vi "Error Checking.vi"(8 "error in (no error)":errorcluster, 11 "VISA resource name":refnum<visa-resource-name>) -> (0 "error out":errorcluster, 2 "Connection Error":bool, 3 "VISA resource name":refnum<visa-resource-name>)   [LabVIEW 2018]
uses:
  <vilib>/Utility/error.llb/DialogType.ctl
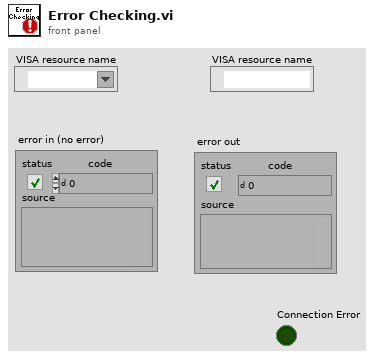
[diagram p1: front panel]
types:
  T1 = typedef "DialogType.ctl" = u16
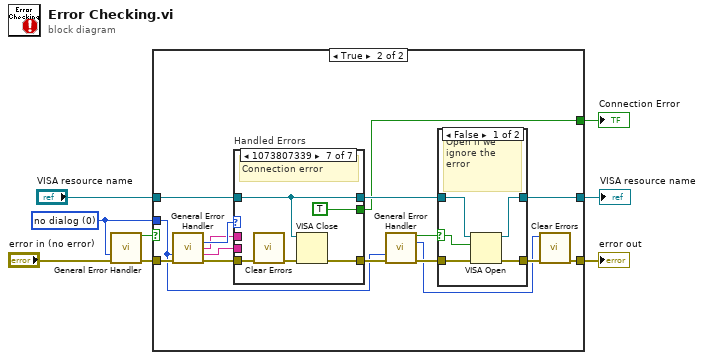
[diagram p0: block diagram]
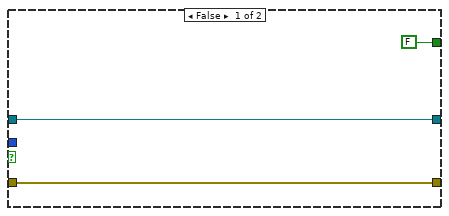
[diagram p2: hidden frame]
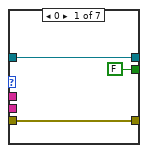
[diagram p4: hidden frame]
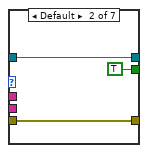
[diagram p5: hidden frame]
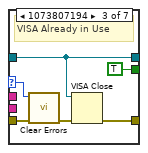
[diagram p6: hidden frame]
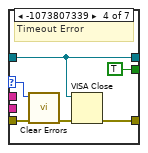
[diagram p7: hidden frame]
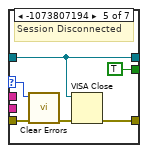
[diagram p8: hidden frame]
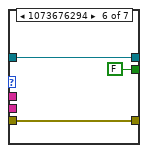
[diagram p9: hidden frame]
diagram:
  w2 = T1 0 items=["no dialog", "OK message", "continue or stop message", "OK message + warnings", "continue/stop + warnings"] ("type of dialog (OK msg:1)")
  n1 = call <vilib>:"General Error Handler.vi"("type of dialog (OK msg:1)"=w2, "error in (no error)"="error in (no error)") -> ("error?"=w8:bool, "error out"=w7:errorcluster)  [unwired: 9 in, 3 out]
  n2 = case shown="True" w8 {
    tunnel: [w11 w26] -> w6
    tunnel: w7 -> [w11 w27]
    tunnel: "VISA resource name" -> [w10 w25]
    tunnel: [w10 w19] -> w3
    tunnel: w2 -> [_ w17]
    tunnel: [FALSE w12] -> w1
    frame False {
    }
    frame True {
      n3 = call <vilib>:"General Error Handler.vi"("type of dialog (OK msg:1)"=w17, "error in (no error)"=w27) -> ("code out"=w15:i32, "source out"=w14:string, "message"=w13:string, "error out"=w24:errorcluster)  [unwired: 9 in, 1 out]
      n4 = case "Handled Errors" shown="1073807339" w15 {
        selector: w15 -> [_ _ w42 w48 w54 _ _]
        tunnel: w24 -> [w37 w40 w44 w50 w56 w61 w65]
        tunnel: [w37 w40 w46 w52 w58 w61 w63] -> w23
        tunnel: w14 -> [_ _ _ _ _ _ _]
        tunnel: w13 -> [_ _ _ _ _ _ _]
        tunnel: w25 -> [w36 w39 w45 w51 w57 w60 w64]
        tunnel: [w36 w39 w45 w51 w57 w60 w64] -> w18
        tunnel: [FALSE TRUE TRUE TRUE TRUE FALSE TRUE] -> w12
        frame 0 {
        }
        frame Default {
        }
        frame 1073807194 {
          # "VISA Already in Use"
          n5 = call <vilib>:"Clear Errors.vi"("error in (no error)"=w44, "specific error code to clear (0: all)"=w42) -> ("error out"=w43:errorcluster)  [unwired: 4 in, 1 out]
          n6 = VISA Close(VISA resource name=w45, error in (no error)=w43) -> (error out=w46:errorcluster)
        }
        frame -1073807339 {
          # "Timeout Error"
          n7 = call <vilib>:"Clear Errors.vi"("error in (no error)"=w50, "specific error code to clear (0: all)"=w48) -> ("error out"=w49:errorcluster)  [unwired: 4 in, 1 out]
          n8 = VISA Close(VISA resource name=w51, error in (no error)=w49) -> (error out=w52:errorcluster)
        }
        frame -1073807194 {
          # "Session Disconnected"
          n9 = call <vilib>:"Clear Errors.vi"("error in (no error)"=w56, "specific error code to clear (0: all)"=w54) -> ("error out"=w55:errorcluster)  [unwired: 4 in, 1 out]
          n10 = VISA Close(VISA resource name=w57, error in (no error)=w55) -> (error out=w58:errorcluster)
        }
        frame 1073676294 {
        }
        frame 1073807339 {
          # "Connection error"
          n11 = call <vilib>:"Clear Errors.vi"("error in (no error)"=w65) -> ("error out"=w66:errorcluster)  [unwired: 5 in, 1 out]
          n12 = VISA Close(VISA resource name=w64, error in (no error)=w66) -> (error out=w63:errorcluster)
        }
      }
      n13 = call <vilib>:"General Error Handler.vi"("type of dialog (OK msg:1)"=w17, "error in (no error)"=w23) -> ("error?"=w22:bool, "code out"=w16:i32, "error out"=w21:errorcluster)  [unwired: 9 in, 2 out]
      n14 = case shown="False" w22 {
        selector: w22 -> [w32 _]
        tunnel: [w29 w34] -> w20
        tunnel: w21 -> [w28 w34]
        tunnel: w18 -> [w31 w33]
        tunnel: [w30 w33] -> w19
        frame False {
          # "Open if we ignore the error"
          n15 = VISA Open(duplicate session (F)=w32, error in (no error)=w28, VISA resource name=w31) -> (VISA resource name=w30:refnum<visa-resource-name>, error out=w29:errorcluster)  [unwired: 2 in]
        }
        frame True {
          # "Leave it closed if we don't ignore"
        }
      }
      n16 = call <vilib>:"Clear Errors.vi"("error in (no error)"=w20, "specific error code to clear (0: all)"=w16) -> ("error out"=w26:errorcluster)  [unwired: 4 in, 1 out]
    }
  }
  "error out" <- w6
  "VISA resource name" <- w3
  "Connection Error" <- w1
